vi "DataTreeCtrl buildDocumentNode.vi"(7 "FileName":string[](array[string]), 9 "Indent":i32, 10 "Root path":path, 11 "Tree Ref In":refnum<vi>) -> (3 "Tree Ref Out":refnum<vi>)   [LabVIEW 2018, in "DataTreeCtrl.lvclass"]
uses:
  DataTreeCtrl.lvclass
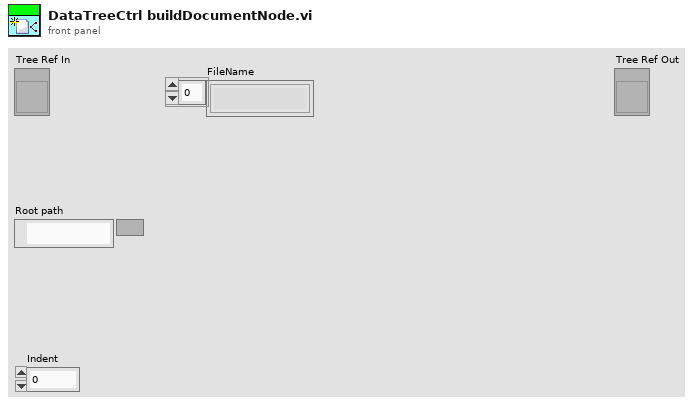
[diagram p1: front panel]
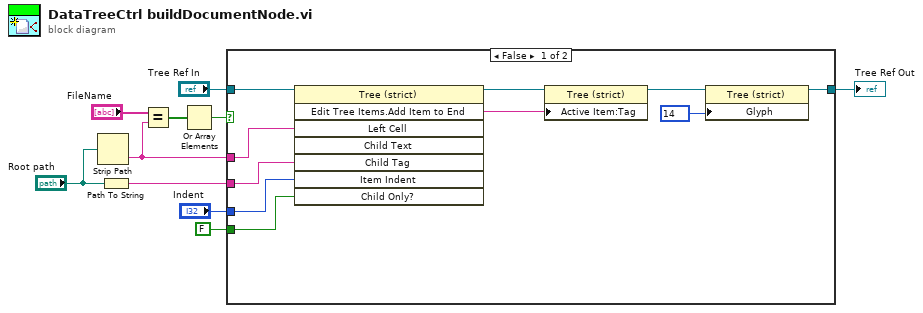
[diagram p0: block diagram]
diagram:
  n1 = Strip Path(path="Root path") -> (name=w3:string)  [unwired: 1 out]
  n2 = Path To String(path="Root path") -> (string=w9:string)
  n3 = Equal?(x="FileName", y=w3) -> (x = y?=w2:bool[])
  n4 = Or Array Elements(Boolean array=w2) -> (logical OR=w1:bool)
  n5 = case shown="False" w1 {
    tunnel: w3 -> [w16 _]
    tunnel: w9 -> [w15 _]
    tunnel: "Tree Ref In" -> [w14 w21]
    tunnel: [w13 w21] -> w7
    tunnel: "Indent" -> [w12 _]
    tunnel: FALSE ("Child Only?") -> [w11 _]
    frame False {
      n6 = invoke class="Tree (strict)" method="Edit Tree Items.Add Item to End"(reference=w14, "Left Cell"=w16, "Child Tag"=w15, "Item Indent"=w12, "Child Only?"=w11) -> (reference out=w20:refnum<vi>, "Edit Tree Items:Add Item to End"=w18:string)  [unwired: 3 in, 6 out]
      n7 = property on="Property Node" class="Tree (strict)"(reference=w20, "Active Item:Tag"=w18) -> (reference out=w19:refnum<vi>)  [unwired: 1 in, 1 out]
      n8 = property class="Tree (strict)"(reference=w19, "Glyph"=14) -> (reference out=w13:refnum<vi>)  [unwired: 1 in, 1 out]
    }
    frame True {
    }
  }
  "Tree Ref Out" <- w7
